vi "GetHeuristicCost.vi"(8 "error in (no error)":errorcluster, 10 "Goal NodeReference":refnum<data-value>, 11 "OccupancyGridMapNode in":refnum<class "NI_Robotics_OccupancyGridMapNode.lvclass">) -> (0 "error out":errorcluster, 2 "hueristic cost":dbl, 3 "OccupancyGridMapNode out":refnum<class "NI_Robotics_OccupancyGridMapNode.lvclass">)   [LabVIEW 2017, in "NI_Robotics_OccupancyGridMapNode.lvclass"]
uses:
  <vilib>/robotics/Navigation/shared/MapNode/OccupancyGridNode/NI_Robotics_OccupancyGridMapNode.lvclass
  <vilib>/robotics/Navigation/shared/MapNode/AbstractMapNode/NI_Robotics_AbstractMapNode.lvclass
  <vilib>/robotics/Navigation/shared/MapNode/OccupancyGridNode/NI_Robotics_OccupancyGridMapNode.lvclass/NI_Robotics_OccupancyGridMapNode.ctl
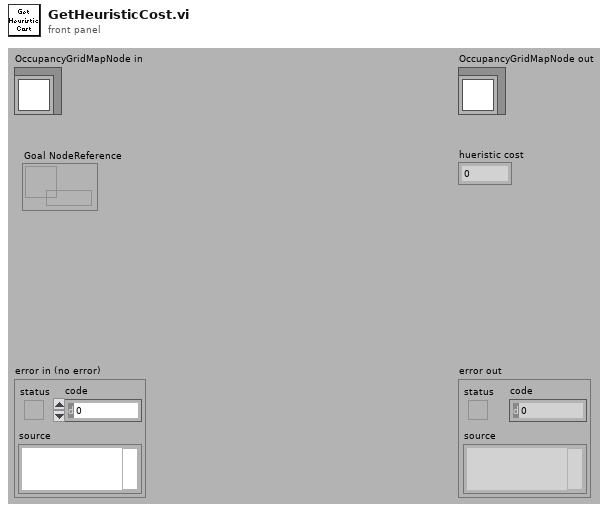
[diagram p1: front panel]
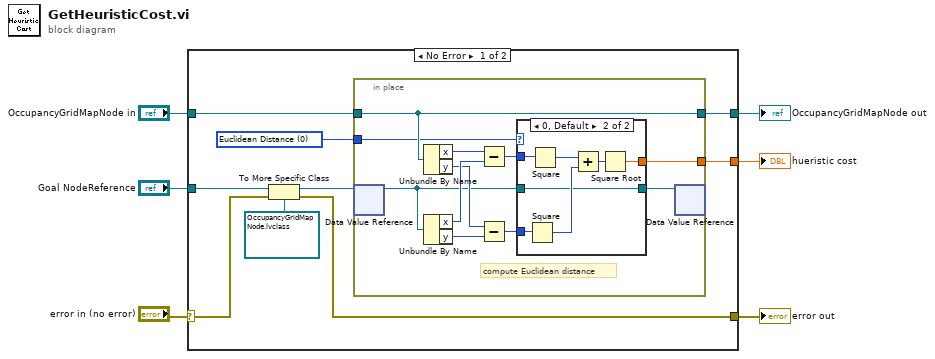
[diagram p0: block diagram]
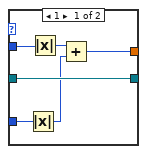
[diagram p2: hidden frame]
diagram:
  n1 = case shown="No Error" "error in (no error)" {
    selector: "error in (no error)" -> [w8 w41]
    tunnel: "OccupancyGridMapNode in" -> [w15 w40]
    tunnel: [w14 w40] -> w5
    tunnel: "Goal NodeReference" -> [w13 _]
    tunnel: [w10 _] -> w3
    tunnel: [w9 w41] -> w2
    frame No Error {
      w7 = u16 0 items=["Euclidean Distance", "Manhattan Distance"] ("heuristic function")
      n2 = To More Specific Class(target class=refnum<data-value> refnum ("data value reference"), reference=w13, error in=w8) -> (specific class reference=w11:refnum<data-value>, error out=w9:errorcluster)
      n3 = in-place {
        in-place-border: w15 -> [w25]
        in-place-border: [w25] -> w14
        in-place-border: [w26] -> w10
        in-place-border: w7 -> [w18]
        # "compute Euclidean distance"
        n4 = in-place-dvr #1(w11) -> (w17:refnum<class "NI_Robotics_OccupancyGridMapNode.lvclass">)  [unwired: 1 out]
        n5 = Unbundle By Name(w25) -> ("x"=w24:i32, "y"=w22:i32)
        n6 = Unbundle By Name(w17) -> ("x"=w23:i32, "y"=w21:i32)
        n7 = Subtract(x=w24, y=w23) -> (x-y=w20:i32)
        n8 = Subtract(x=w22, y=w21) -> (x-y=w19:i32)
        n9 = case shown="0, Default" w18 {
          tunnel: [w27 w39] -> w26
          tunnel: w20 -> [w32 w38]
          tunnel: w19 -> [w31 w37]
          tunnel: w17 -> [w30 w33]
          tunnel: [w30 w33] -> w16
          frame 1 {
            n10 = Absolute Value(x=w31) -> (abs(x)=w28:i32)
            n11 = Absolute Value(x=w32) -> (abs(x)=w29:i32)
            n12 = Add(x=w29, y=w28) -> (x+y=w27:i32)
          }
          frame 0, Default {
            n13 = Square(x=w37) -> (x^2=w35:i32)
            n14 = Square(x=w38) -> (x^2=w36:i32)
            n15 = Add(x=w36, y=w35) -> (x+y=w34:i32)
            n16 = Square Root(x=w34) -> (sqrt(x)=w39:dbl)
          }
        }
        n17 = in-place-dvr #1(w16) -> ()  [unwired: 2 out]
      }
    }
    frame Error {
    }
  }
  "error out" <- w2
  "OccupancyGridMapNode out" <- w5
  "hueristic cost" <- w3
